vi "Translator.CleanupControls.vi"(8 "error in":errorcluster, 10 "Controls":T1[](array[typedef]), 11 "VI ref in":refnum<vi>) -> (0 "error out":errorcluster, 3 "VI ref out":refnum<vi>)   [LabVIEW 2019, in "Tools.lvlib"]
uses:
  Tools.lvlib
  Translator.ControlData.ctl
  Translator.ControlTypes.ctl
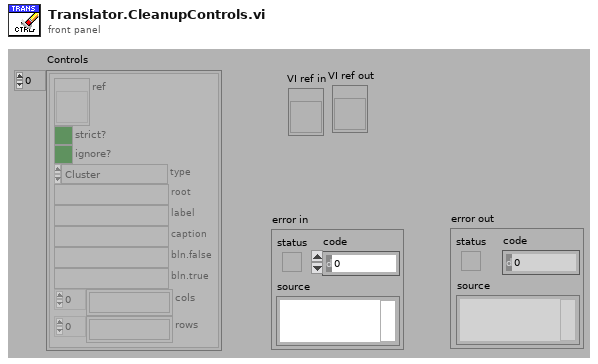
[diagram p1: front panel]
types:
  T1 = typedef "Tools.lvlib/Translator.ControlData.ctl" = cluster{"ref":refnum<vi>, "strict?":bool, "ignore?":bool, "type":T2, "root":string, "label":string, "caption":string, "bln.false":string, "bln.true":string, "cols":string[], "rows":string[]}
  T2 = typedef "Tools.lvlib/Translator.ControlTypes.ctl" = enum16{"Cluster", "Array", "Boolean", "Ring", "String", "Tab", "Listbox", "Multicolumn listbox", "Table", "Other"}
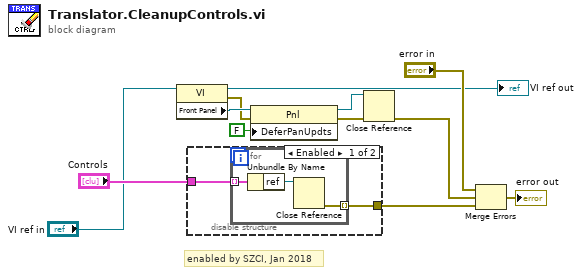
[diagram p0: block diagram]
diagram:
  # "enabled by SZCI, Jan 2018"
  n1 = property class="VI"(reference="VI ref in") -> (reference out=→"VI ref out":refnum<vi>, error out=w8:errorcluster, "Front Panel"=w9:refnum<vi>)  [unwired: 1 in]
  n2 = disable-structure shown="Enabled" {
    disable-tunnel: "Controls" -> [w14 _]
    disable-tunnel: [w13 _] -> w11
    frame Enabled {
      n3 = for {
        tunnel: w14 -> [w17] mode=indexing
        tunnel: [w15] -> w13 mode=indexing
        n4 = Unbundle By Name(w17) -> ("ref"=w16:refnum<vi>)
        n5 = Close Reference(reference=w16) -> (error out=w15:errorcluster)  [unwired: 1 in]
      }
    }
    frame Disabled {
    }
  }
  n6 = property class="Pnl"(reference=w9, error in=w8, "DeferPanUpdts"=FALSE ("Defer Panel Updates")) -> (reference out=w5:refnum<vi>, error out=w6:errorcluster)
  n7 = Close Reference(reference=w5, error in (no error)=w6) -> (error out=w2:errorcluster)
  n8 = Merge Errors("error in", w2, w11) -> (→"error out":errorcluster)
